vi "String - Key Down.vi"(8 "error in (no error)":errorcluster, 10 "VKey":T1, 11 "Loop data in":T2={"Config"={"List"=[], "max rows"=8, "Listbox placement"=enum."None", "String Color Options"={"Use? (F)"=FALSE, "Color - Valid"=0, "Color - Invalid"=0, "Allow blank?"=FALSE}}, "Refs"={"String"=refnum, "Listbox"=refnum}, "State"={"LB active?"=FALSE}}) -> (0 "error out":errorcluster, 3 "Loop data out":T2={"Config"={"List"=[], "max rows"=8, "Listbox placement"=enum."None", "String Color Options"={"Use? (F)"=FALSE, "Color - Valid"=0, "Color - Invalid"=0, "Allow blank?"=FALSE}}, "Refs"={"String"=refnum, "Listbox"=refnum}, "State"={"LB active?"=FALSE}})   [LabVIEW 2021, in "Autocomplete Textbox.lvlib"]
uses:
  Autocomplete Textbox.lvlib
  Loop Data.ctl
  Inputs.ctl
  Classes/Handle/Listbox placement.ctl
  Color String Options.ctl
  Refs.ctl
  State data.ctl
  <vilib>/event_ctls.llb/eventvkey.ctl
  Classes/Handle/Handle.lvclass
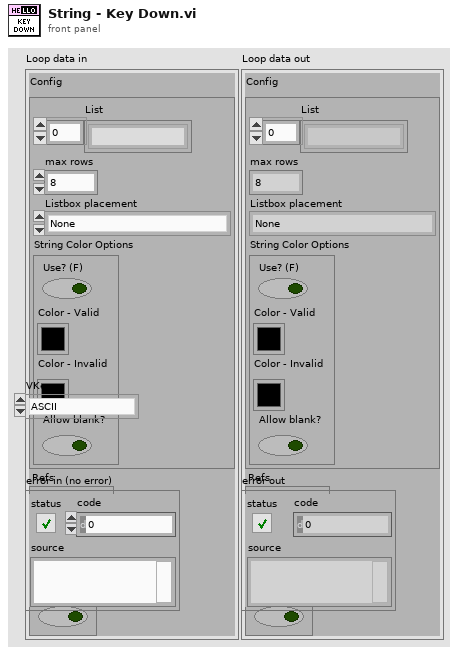
[diagram p1: front panel]
types:
  T1 = typedef "eventvkey.ctl" = enum16{"ASCII", "Enter", "Return", "Shift", "Ctrl", "Alt", "Cmd", "Opt", "Caps", "NumLock", "Clear", "Break", "Up", "Down", "Left", "Right", "Insert", "Delete", "Home", "End", "PageUp", "PageDown", "Escape", "Help", "Pause", "ScrollLock", "F1", "F2", "F3", "F4", "F5", "F6", "F7", "F8", "F9", "F10", "F11", "F12", "F13", "F14", "F15", "F16", "F17", "F18", "F19", "F20", "F21", "F22", "F23", "F24", "Play", "VolumeUp", "VolumeDown", "Mute", "Two Byte Char"}
  T2 = typedef "Autocomplete Textbox.lvlib/Loop Data.ctl" = cluster{"Config":T3, "Refs":T6, "State":T7}
  T3 = typedef "Autocomplete Textbox.lvlib/Inputs.ctl" = cluster{"List":string[], "max rows":i32, "Listbox placement":T4, "String Color Options":T5}
  T4 = typedef "Autocomplete Textbox.lvlib/Handle.lvclass/Listbox placement.ctl" = enum16{"None", "Under String", "Fit to Pane"}
  T5 = typedef "Autocomplete Textbox.lvlib/Color String Options.ctl" = cluster{"Use? (F)":bool, "Color - Valid":u32, "Color - Invalid":u32, "Allow blank?":bool}
  T6 = typedef "Autocomplete Textbox.lvlib/Refs.ctl" = cluster{"String":refnum<vi>, "Listbox":refnum<vi>}
  T7 = typedef "Autocomplete Textbox.lvlib/State data.ctl" = cluster{"LB active?":bool}
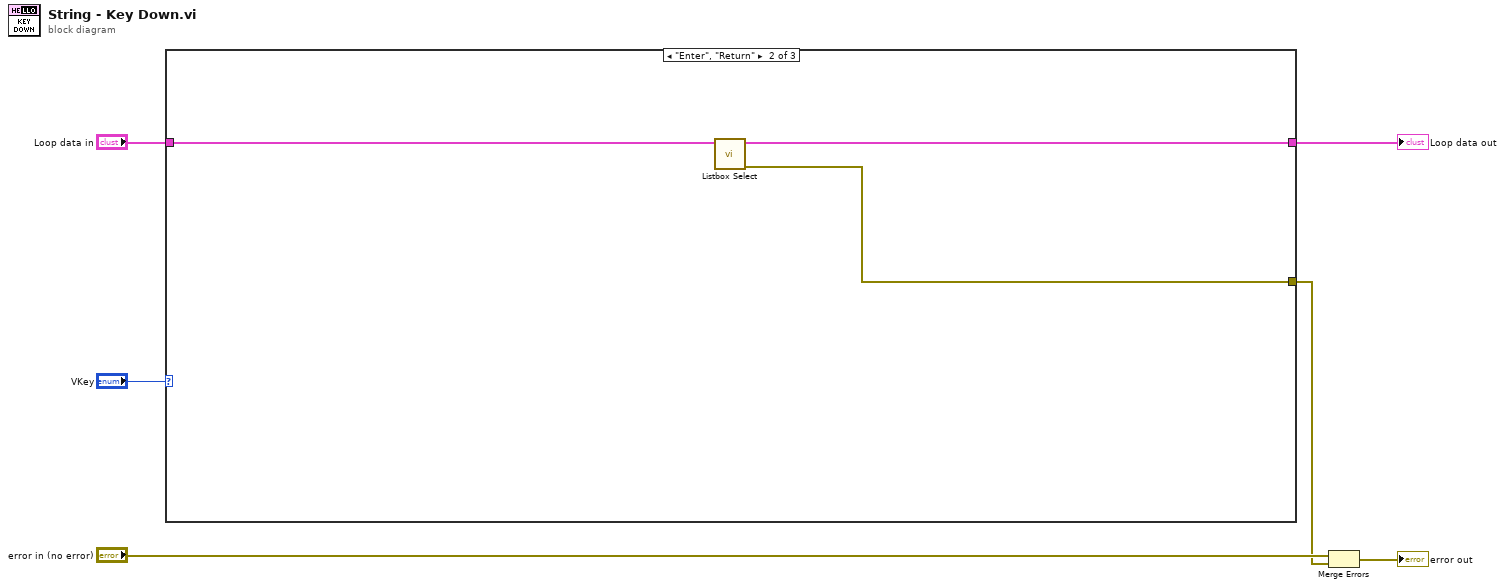
[diagram p0: block diagram]
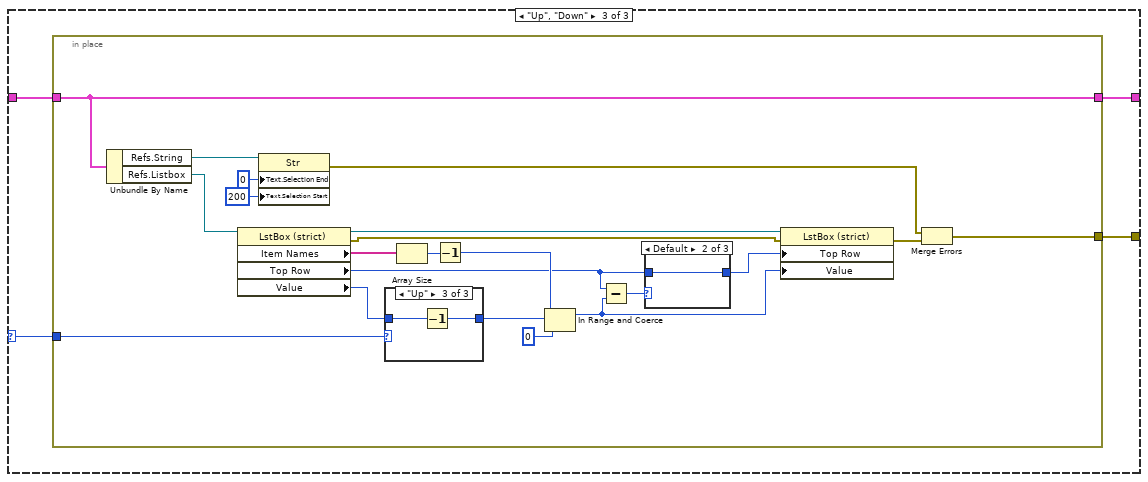
[diagram p3: hidden frame]
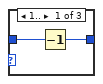
[diagram p4: hidden frame]
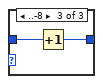
[diagram p5: hidden frame]
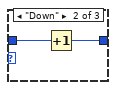
[diagram p7: hidden frame]
diagram:
  n1 = case shown="\"Enter\", \"Return\"" "VKey" {
    selector: "VKey" -> [_ _ w14]
    tunnel: [_ w10 w13] -> w3
    tunnel: "Loop data in" -> [w7 w9 w12]
    tunnel: [w7 w8 w11] -> w1
    frame Default {
    }
    frame "Enter", "Return" {
      n2 = call "Listbox Select.vi"("Loop data in"=w9) -> ("error out"=w10:errorcluster, "Loop data out"=w8:T2)  [unwired: 9 in]
    }
    frame "Up", "Down" {
      n3 = in-place {
        in-place-border: w14 -> [w32]
        in-place-border: [w16] -> w13
        in-place-border: w12 -> [w15]
        in-place-border: [w15] -> w11
        n4 = Unbundle By Name(w15) -> ("Refs.String"=w20:refnum<vi>, "Refs.Listbox"=w21:refnum<vi>)
        n5 = property class="LstBox (strict)"(reference=w21) -> (reference out=w34:refnum<vi>, error out=w19:errorcluster, "Item Names"=w31:string[], "Top Row"=w23:i32, "Value"=w26:i32)  [unwired: 1 in]
        n6 = property class="Str"(reference=w20, "Text.Selection End"=u32 0 ("Text.Selection:End"), "Text.Selection Start"=u32 200 ("Text.Scroll Position")) -> (error out=w17:errorcluster)  [unwired: 1 in, 1 out]
        n7 = case shown="\"Up\"" w32 {
          tunnel: w26 -> [_ w42 w44]
          tunnel: [_ w41 w43] -> w33
          frame Default {
          }
          frame "Down" {
            n8 = Increment(x=w42) -> (x+1=w41:i32)
          }
          frame "Up" {
            n9 = Decrement(x=w44) -> (x-1=w43:i32)
          }
        }
        n10 = Array Size(array=w31) -> (size(s)=w30:i32)
        n11 = Decrement(x=w30) -> (x-1=w29:i32)
        n12 = In Range and Coerce(upper limit=w29, x=w33, lower limit=0) -> (coerced(x)=w24:i32)  [unwired: 1 out]
        n13 = Subtract(x=w23, y=w24) -> (x-y=w25:i32)
        n14 = case shown="Default" w25 {
          tunnel: w23 -> [w37 w38 w40]
          tunnel: [w36 w38 w39] -> w22
          frame 1.. {
            n15 = Decrement(x=w37) -> (x-1=w36:i32)
          }
          frame Default {
          }
          frame ..-8 {
            n16 = Increment(x=w40) -> (x+1=w39:i32)
          }
        }
        n17 = property class="LstBox (strict)"(reference=w34, error in=w19, "Top Row"=w22, "Value"=w24) -> (error out=w18:errorcluster)  [unwired: 1 out]
        n18 = Merge Errors(w17, w18) -> (w16:errorcluster)
      }
    }
  }
  "Loop data out" <- w1
  n19 = Merge Errors("error in (no error)", w3) -> (→"error out":errorcluster)
